vi "Implode String.vi"(7 "Delim (comma)":string=",", 11 "String Array":string[](array[string])) -> (3 "String":string)   [LabVIEW 2020, in "Stream.lvlib"]
uses:
  Stream.lvlib
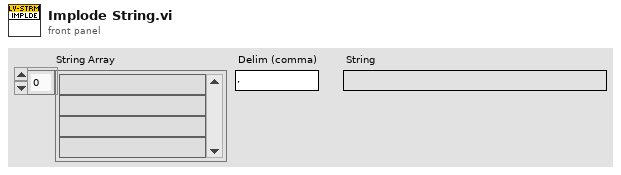
[diagram p1: front panel]
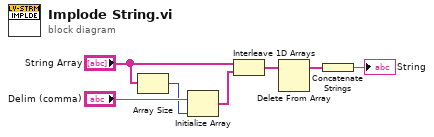
[diagram p0: block diagram]
diagram:
  n1 = Array Size(array="String Array") -> (size(s)=w1:i32)
  n2 = Initialize Array("Delim (comma)", w1) -> (w5:string[])
  n3 = Interleave 1D Arrays("String Array", w5) -> (w3:string[])
  n4 = Delete From Array(array=w3) -> (array with subset deleted=w2:string[])  [unwired: 2 in, 1 out]
  n5 = Concatenate Strings(w2) -> (→"String":string)
